vi "Read Log File Path.vi"(8 "error in (no error)":errorcluster, 11 "File Sink in":refnum<class "File Sink.lvclass">) -> (0 "error out":errorcluster, 2 "Log File Path":path, 3 "File Sink out":refnum<class "File Sink.lvclass">)   [LabVIEW 2020, in "LV Log.lvlib" / "File Sink.lvclass"]
uses:
  File Sink.lvclass
  File Sink.lvclass/File Sink.ctl
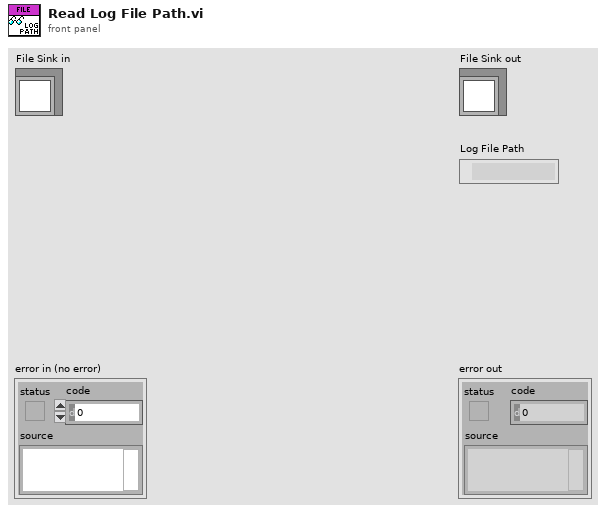
[diagram p1: front panel]
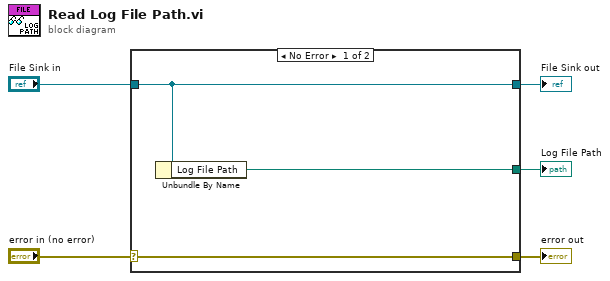
[diagram p0: block diagram]
diagram:
  n1 = case shown="No Error" "error in (no error)" {
    selector: "error in (no error)" -> [w8 w9]
    tunnel: [w8 w9] -> w4
    tunnel: [w7 w10] -> w2
    tunnel: "File Sink in" -> [w7 w10]
    tunnel: [w6 _] -> w1
    frame No Error {
      n2 = Unbundle By Name(w7) -> ("Log File Path"=w6:path)
    }
    frame Error {
    }
  }
  "error out" <- w4
  "File Sink out" <- w2
  "Log File Path" <- w1
